vi "Close Log.vi"(8 "error in":errorcluster) -> (0 "error out":errorcluster)   [LabVIEW 2015, in "Logger.lvlib"]
uses:
  Logger.lvlib
  support/Message Queue/Message Queue.lvlib
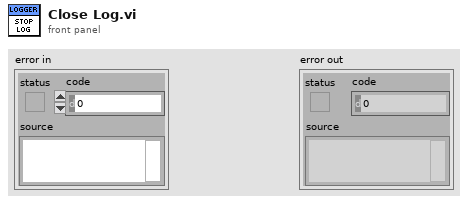
[diagram p1: front panel]
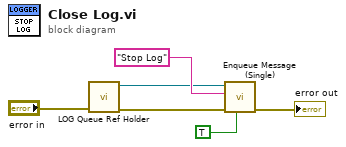
[diagram p0: block diagram]
diagram:
  n1 = call "LOG Queue Ref Holder.vi"("error in"="error in") -> ("error out"=w2:errorcluster, "Input Message Queue"=w3:refnum<queue>)  [unwired: 9 in]
  n2 = call "Enqueue Message (Single).vi"("Priority Message? (F)"=TRUE, "error in (no error)"=w2, "Message"="Stop Log", "Message Queue"=w3) -> ("error out"=→"error out":errorcluster)  [unwired: 6 in, 1 out]
